vi "Read DVM.vi"(8 "error in (no error)":errorcluster, 11 "VISA resource name":refnum<visa-resource-name>) -> (0 "error out":errorcluster, 2 "Measured DVM Voltage (V)":dbl format="%.3f", 3 "VISA resource name out":refnum<visa-resource-name>)   [LabVIEW 2021, in "BK Precision 9200 Series.lvlib"]
doc: "Reads the measured voltage from the built-in DVM of the instrument."
uses:
  <instrlib>/BK Precision 9200 Series/BK Precision 9200 Series.lvlib
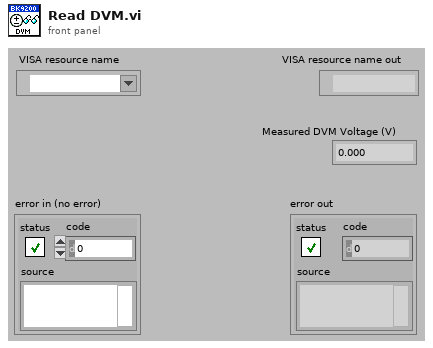
[diagram p1: front panel]
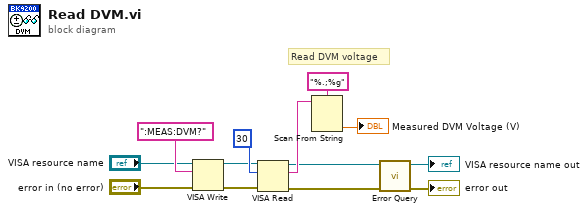
[diagram p0: block diagram]
diagram:
  # "Read DVM voltage"
  n1 = VISA Write(VISA resource name="VISA resource name", write buffer=":MEAS:DVM?", error in (no error)="error in (no error)") -> (VISA resource name out=w9:refnum<visa-resource-name>, error out=w8:errorcluster)  [unwired: 1 out]
  n2 = VISA Read(VISA resource name=w9, byte count=30, error in (no error)=w8) -> (VISA resource name out=w3:refnum<visa-resource-name>, read buffer=w6:string, error out=w2:errorcluster)  [unwired: 1 out]
  n3 = Scan From String(format string="%.;%g", input string=w6) -> (output 1=→"Measured DVM Voltage (V)":dbl)  [unwired: 3 in, 3 out]
  n4 = call <instrlib>:"Error Query.vi"("error in (no error)"=w2, "VISA resource name"=w3) -> ("error out"=→"error out":errorcluster, "VISA resource name out"=→"VISA resource name out":refnum<visa-resource-name>)  [unwired: 6 in, 2 out]
